vi "minimal.vi"(6 "Numeric":dbl, 9 "Array":dbl[](array[numeric]), 11 "Array 2":dbl[][](array[numeric])) -> (3 "Numeric 2":dbl)   [LabVIEW 2018]
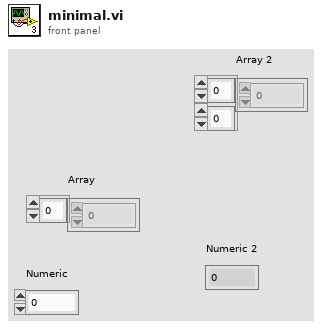
[diagram p1: front panel]
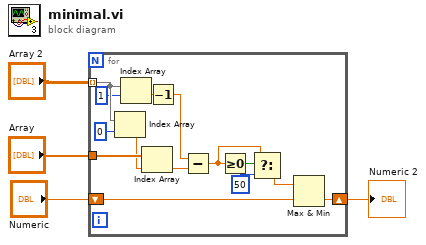
[diagram p0: block diagram]
diagram:
  n1 = for {
    tunnel: "Array 2" -> [w18] mode=indexing
    tunnel: "Array" -> [w15]
    shift-right: [w12] -> w2
    shift-left: "Numeric" -> [w11]
    n2 = Index Array(array=w18, index=0) -> (element=w14:dbl)
    n3 = Index Array(array=w18, index=1) -> (element=w13:dbl)
    n4 = Index Array(array=w15, index=w14) -> (element=w9:dbl)
    n5 = Decrement(x=w13) -> (x-1=w10:dbl)
    n6 = Subtract(x=w10, y=w9) -> (x-y=w5:dbl)
    n7 = Greater Or Equal To 0?(x=w5) -> (x >= 0?=w8:bool)
    n8 = Select(t=w5, s=w8, f=50) -> (s? t:f=w6:dbl)
    n9 = Max & Min(x=w6, y=w11) -> (min(x,y)=w12:dbl)  [unwired: 1 out]
  }
  "Numeric 2" <- w2
